vi "Arduino read multiple 11-08-2017 w median filt.vi"(7 "loop cycle in":u32=300, 8 "freq in":dbl[](array[numeric]), 10 "arduino addresses in":T2) -> (0 "loop cycle out":u32=300, 1 "freq out":dbl[](array[numeric]), 3 "arduino addresses out":T1)   [LabVIEW 2014]
uses:
  <vilib>/Analysis/NI_AALBase.lvlib
panel:
  out "median":dbl format="%0.2f"
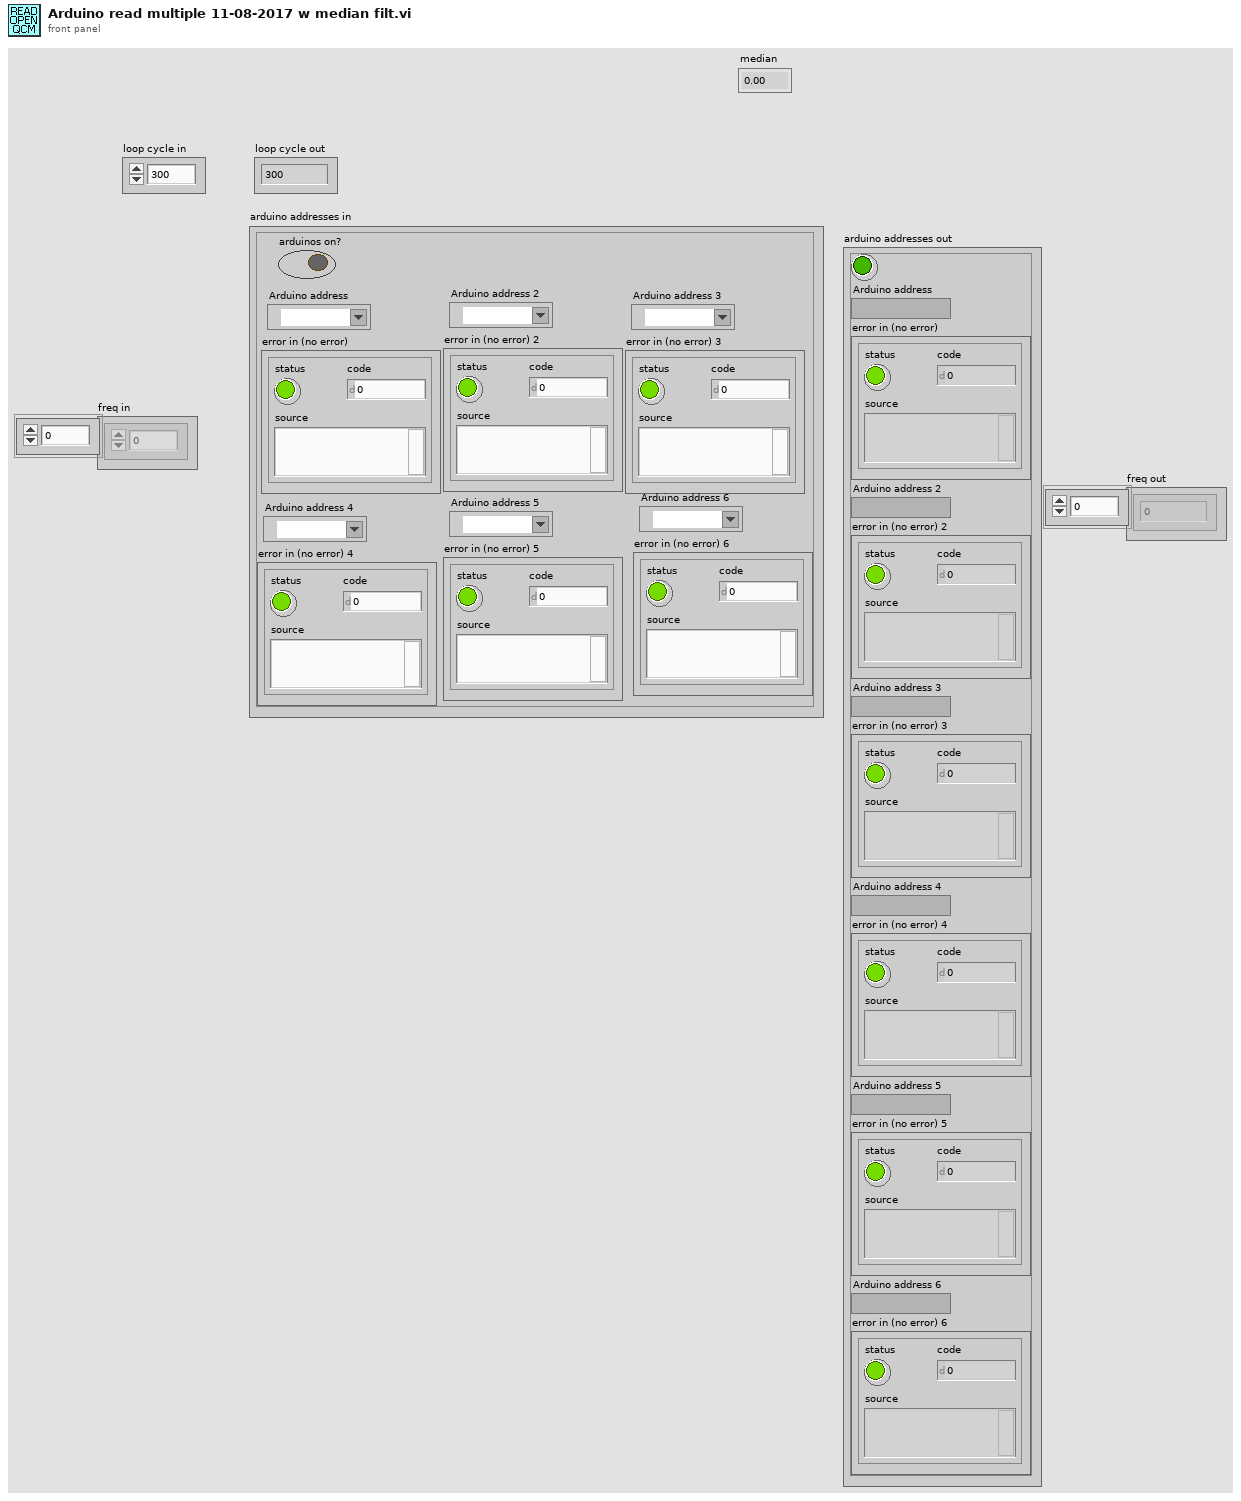
[diagram p1: front panel]
types:
  T1 = cluster{"Boolean":bool, "Arduino address":refnum<visa-resource-name>, "error in (no error)":errorcluster, "Arduino address 2":refnum<visa-resource-name>, "error in (no error) 2":errorcluster, "Arduino address 3":refnum<visa-resource-name>, "error in (no error) 3":errorcluster, "Arduino address 4":refnum<visa-resource-name>, "error in (no error) 4":errorcluster, "Arduino address 5":refnum<visa-resource-name>, "error in (no error) 5":errorcluster, "Arduino address 6":refnum<visa-resource-name>, "error in (no error) 6":errorcluster}
  T2 = cluster{"Arduino address":refnum<visa-resource-name>, "error in (no error)":errorcluster, "Arduino address 2":refnum<visa-resource-name>, "error in (no error) 2":errorcluster, "Arduino address 3":refnum<visa-resource-name>, "error in (no error) 3":errorcluster, "Arduino address 4":refnum<visa-resource-name>, "error in (no error) 4":errorcluster, "Arduino address 5":refnum<visa-resource-name>, "error in (no error) 5":errorcluster, "Arduino address 6":refnum<visa-resource-name>, "error in (no error) 6":errorcluster, "arduinos on?":bool}
  T3 = cluster{bool, "Arduino address":refnum<visa-resource-name>, "error in (no error)":errorcluster, "Arduino address 2":refnum<visa-resource-name>, "error in (no error) 2":errorcluster, "Arduino address 3":refnum<visa-resource-name>, "error in (no error) 3":errorcluster, "Arduino address 4":refnum<visa-resource-name>, "error in (no error) 4":errorcluster, "Arduino address 5":refnum<visa-resource-name>, "error in (no error) 5":errorcluster, "Arduino address 6":refnum<visa-resource-name>, "error in (no error) 6":errorcluster}
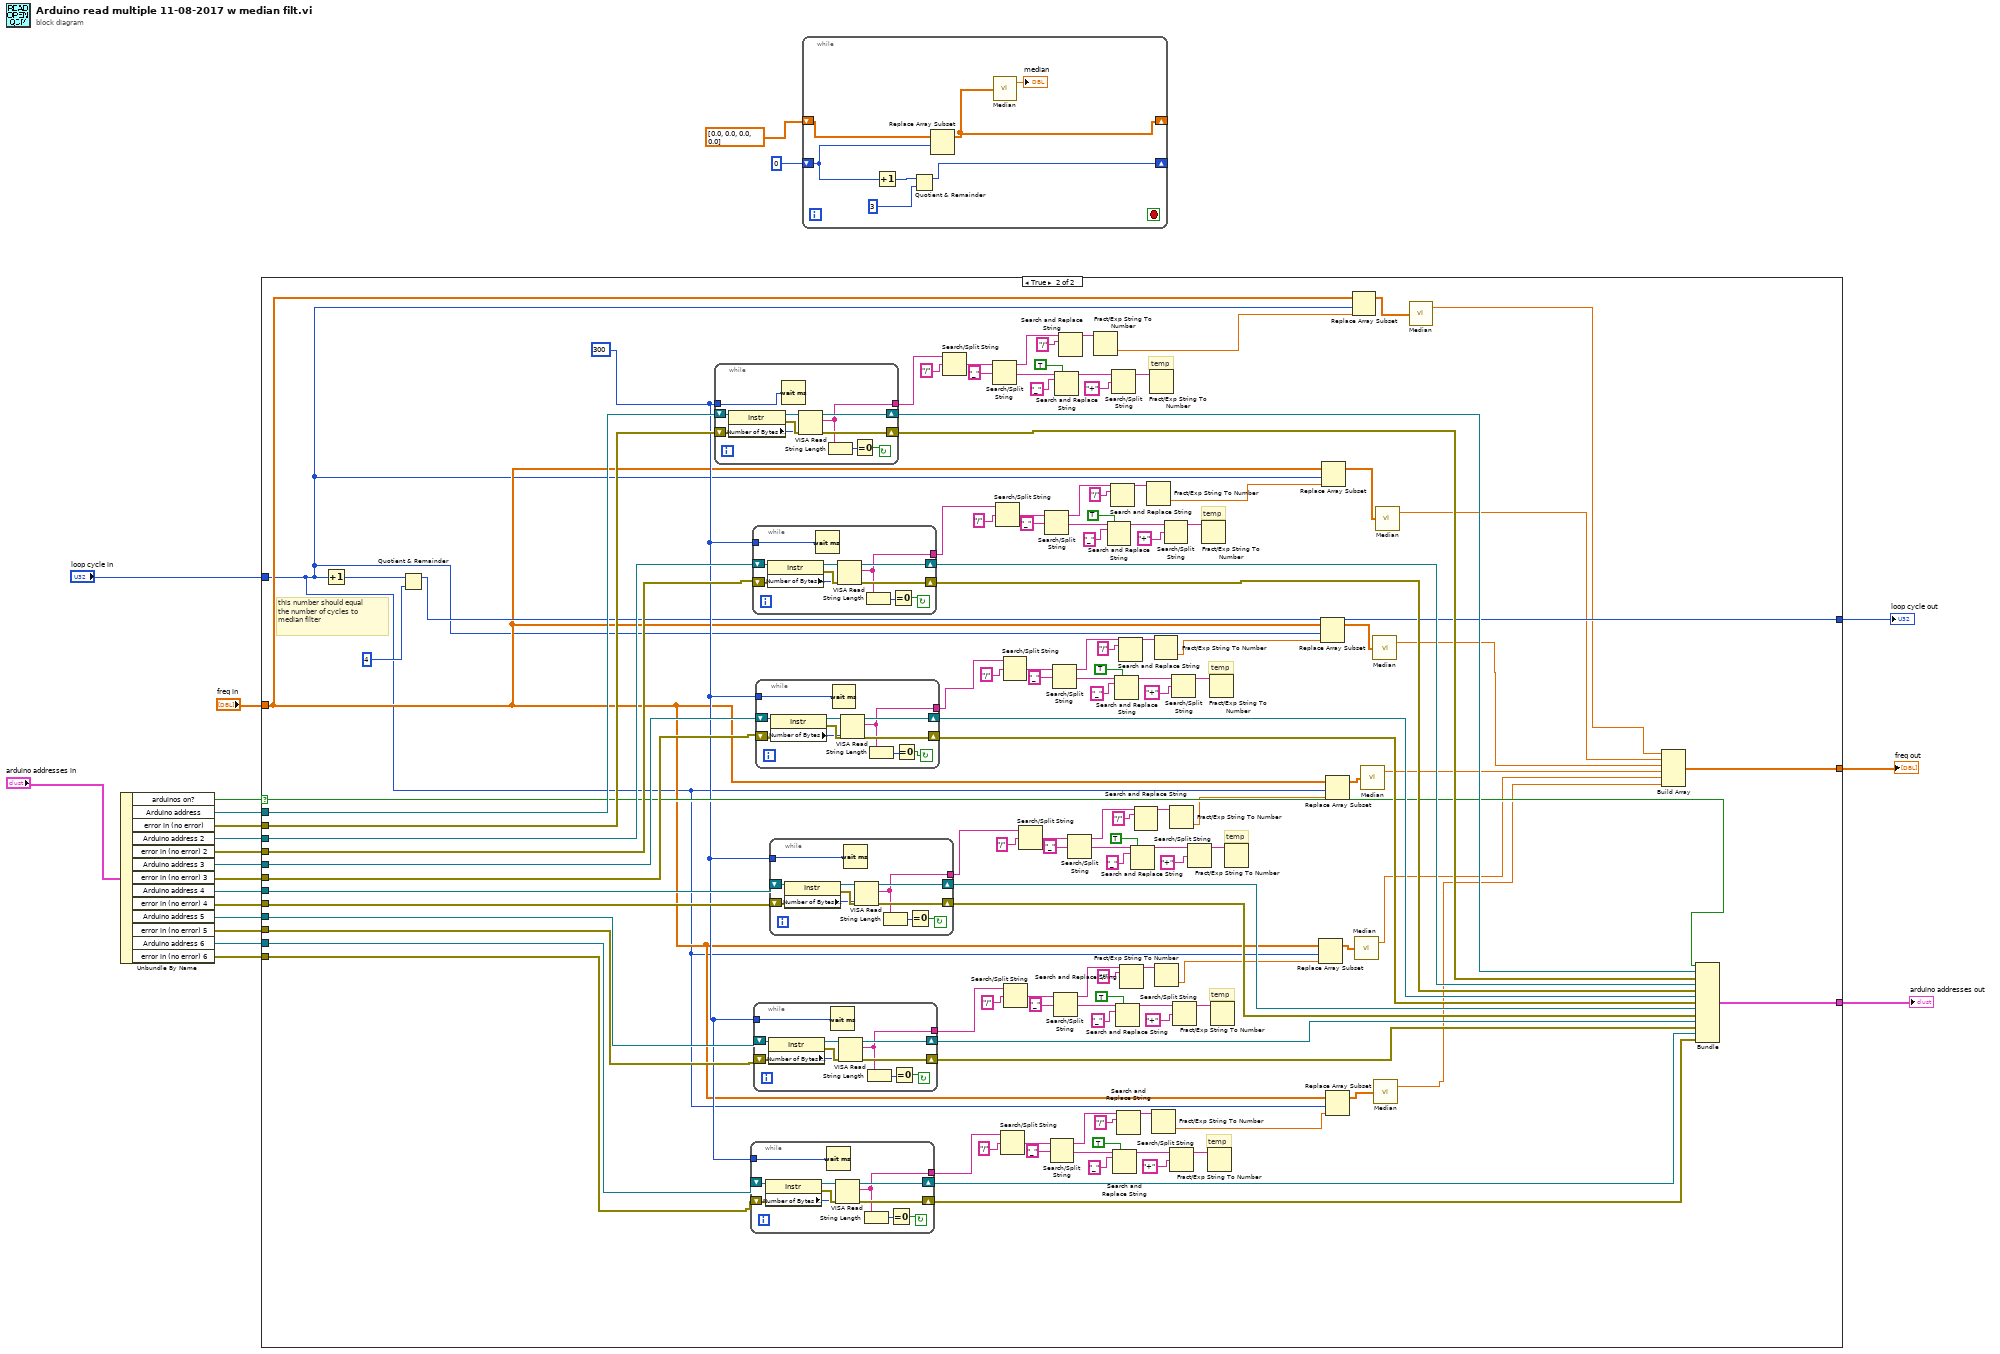
[diagram p0: block diagram]
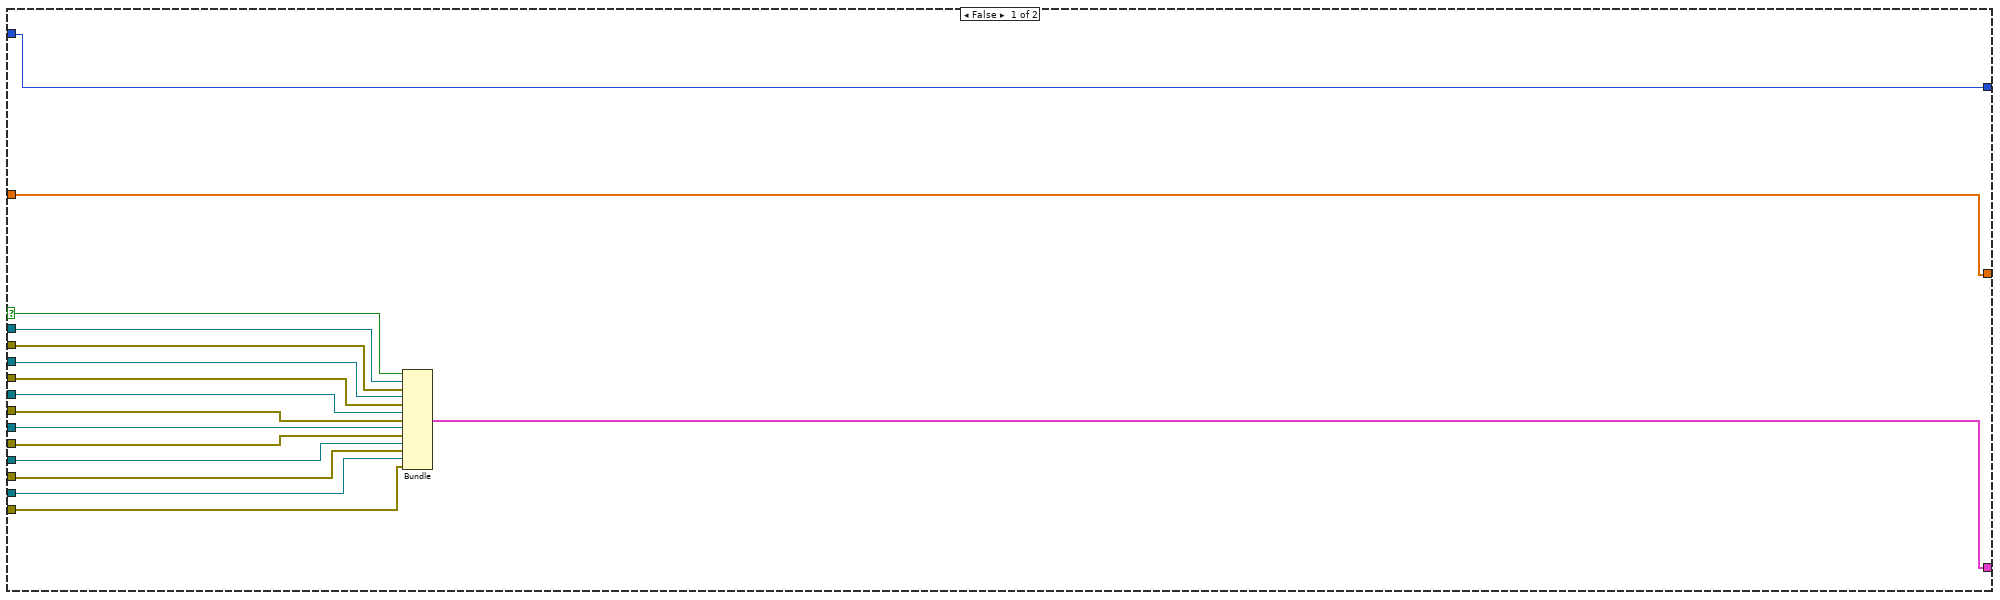
[diagram p2: hidden frame]
diagram:
  n1 = Unbundle By Name("arduino addresses in") -> ("arduinos on?"=w21:bool, "Arduino address"=w20:refnum<visa-resource-name>, "error in (no error)"=w19:errorcluster, "Arduino address 2"=w18:refnum<visa-resource-name>, "error in (no error) 2"=w17:errorcluster, "Arduino address 3"=w16:refnum<visa-resource-name>, "error in (no error) 3"=w15:errorcluster, "Arduino address 4"=w13:refnum<visa-resource-name>, "error in (no error) 4"=w12:errorcluster, "Arduino address 5"=w11:refnum<visa-resource-name>, "error in (no error) 5"=w10:errorcluster, "Arduino address 6"=w9:refnum<visa-resource-name>, "error in (no error) 6"=w8:errorcluster)
  n2 = case shown="True" w21 {
    selector: w21 -> [w37 w64]
    tunnel: [w22 w63] -> w7
    tunnel: w20 -> [w36 w76]
    tunnel: w19 -> [w35 w75]
    tunnel: w18 -> [w34 w74]
    tunnel: w17 -> [w33 w73]
    tunnel: w16 -> [w32 w72]
    tunnel: w15 -> [w31 w71]
    tunnel: w13 -> [w30 w70]
    tunnel: w12 -> [w29 w69]
    tunnel: w11 -> [w28 w68]
    tunnel: w10 -> [w27 w67]
    tunnel: w9 -> [w26 w66]
    tunnel: w8 -> [w25 w65]
    tunnel: [w23 w62] -> w6
    tunnel: "freq in" -> [w23 w57]
    tunnel: "loop cycle in" -> [w24 w56]
    tunnel: [w24 w58] -> w3
    frame False {
      n3 = Bundle(w37, "Arduino address"=w36, "error in (no error)"=w35, "Arduino address 2"=w34, "error in (no error) 2"=w33, "Arduino address 3"=w32, "error in (no error) 3"=w31, "Arduino address 4"=w30, "error in (no error) 4"=w29, "Arduino address 5"=w28, "error in (no error) 5"=w27, "Arduino address 6"=w26, "error in (no error) 6"=w25) -> (w22:T3)  [unwired: 1 in]
    }
    frame True {
      w61 = u32 300 ("milliseconds to wait")
      # "this number should equal the number of cycles to median filter"
      # "temp"
      # "temp"
      # "temp"
      # "temp"
      # "temp"
      # "temp"
      n4 = Increment(x=w56) -> (x+1=w59:u32)
      n5 = Quotient & Remainder(x=w59, y=u32 4 ("this number should equal the nubmer of cycles to take median over")) -> (x-y*floor(x/y)=w58:u32)  [unwired: 1 out]
      n6 = while {
        shift-right: [w232] -> w88
        shift-left: w76 -> [w230]
        shift-right: [w231] -> w87
        shift-left: w75 -> [w229]
        tunnel: [w223] -> w154
        tunnel: w61 -> [w222]
        stop <- w224 continue-if-true
        n7 = property class="Instr"(reference=w230, error in=w229) -> (reference out=w227:refnum<visa-resource-name>, error out=w228:errorcluster, "Serial Settings:Number of Bytes at Serial Port"=w226:u32)
        n8 = Wait (ms)(milliseconds to wait=w222) -> ()  [unwired: 1 out]
        n9 = VISA Read(VISA resource name=w227, byte count=w226, error in (no error)=w228) -> (VISA resource name out=w232:refnum<visa-resource-name>, read buffer=w223:string, error out=w231:errorcluster)  [unwired: 1 out]
        n10 = String Length(string=w223) -> (length=w225:i32)
        n11 = Equal To 0?(x=w225) -> (x = 0?=w224:bool)
      }
      n12 = while {
        shift-right: [w177] -> w79
        shift-left: w66 -> [w175]
        shift-right: [w176] -> w78
        shift-left: w65 -> [w174]
        tunnel: [w168] -> w89
        tunnel: w61 -> [w167]
        stop <- w169 continue-if-true
        n13 = property class="Instr"(reference=w175, error in=w174) -> (reference out=w172:refnum<visa-resource-name>, error out=w173:errorcluster, "Serial Settings:Number of Bytes at Serial Port"=w171:u32)
        n14 = Wait (ms)(milliseconds to wait=w167) -> ()  [unwired: 1 out]
        n15 = VISA Read(VISA resource name=w172, byte count=w171, error in (no error)=w173) -> (VISA resource name out=w177:refnum<visa-resource-name>, read buffer=w168:string, error out=w176:errorcluster)  [unwired: 1 out]
        n16 = String Length(string=w168) -> (length=w170:i32)
        n17 = Equal To 0?(x=w170) -> (x = 0?=w169:bool)
      }
      n18 = while {
        shift-right: [w221] -> w86
        shift-left: w74 -> [w219]
        shift-right: [w220] -> w85
        shift-left: w73 -> [w218]
        tunnel: [w212] -> w141
        tunnel: w61 -> [w211]
        stop <- w213 continue-if-true
        n19 = property class="Instr"(reference=w219, error in=w218) -> (reference out=w216:refnum<visa-resource-name>, error out=w217:errorcluster, "Serial Settings:Number of Bytes at Serial Port"=w215:u32)
        n20 = Wait (ms)(milliseconds to wait=w211) -> ()  [unwired: 1 out]
        n21 = VISA Read(VISA resource name=w216, byte count=w215, error in (no error)=w217) -> (VISA resource name out=w221:refnum<visa-resource-name>, read buffer=w212:string, error out=w220:errorcluster)  [unwired: 1 out]
        n22 = String Length(string=w212) -> (length=w214:i32)
        n23 = Equal To 0?(x=w214) -> (x = 0?=w213:bool)
      }
      n24 = while {
        shift-right: [w188] -> w77
        shift-left: w68 -> [w186]
        shift-right: [w187] -> w80
        shift-left: w67 -> [w185]
        tunnel: [w179] -> w102
        tunnel: w61 -> [w178]
        stop <- w180 continue-if-true
        n25 = property class="Instr"(reference=w186, error in=w185) -> (reference out=w183:refnum<visa-resource-name>, error out=w184:errorcluster, "Serial Settings:Number of Bytes at Serial Port"=w182:u32)
        n26 = Wait (ms)(milliseconds to wait=w178) -> ()  [unwired: 1 out]
        n27 = VISA Read(VISA resource name=w183, byte count=w182, error in (no error)=w184) -> (VISA resource name out=w188:refnum<visa-resource-name>, read buffer=w179:string, error out=w187:errorcluster)  [unwired: 1 out]
        n28 = String Length(string=w179) -> (length=w181:i32)
        n29 = Equal To 0?(x=w181) -> (x = 0?=w180:bool)
      }
      n30 = while {
        shift-right: [w210] -> w84
        shift-left: w72 -> [w208]
        shift-right: [w209] -> w83
        shift-left: w71 -> [w207]
        tunnel: [w201] -> w128
        tunnel: w61 -> [w200]
        stop <- w202 continue-if-true
        n31 = property class="Instr"(reference=w208, error in=w207) -> (reference out=w205:refnum<visa-resource-name>, error out=w206:errorcluster, "Serial Settings:Number of Bytes at Serial Port"=w204:u32)
        n32 = Wait (ms)(milliseconds to wait=w200) -> ()  [unwired: 1 out]
        n33 = VISA Read(VISA resource name=w205, byte count=w204, error in (no error)=w206) -> (VISA resource name out=w210:refnum<visa-resource-name>, read buffer=w201:string, error out=w209:errorcluster)  [unwired: 1 out]
        n34 = String Length(string=w201) -> (length=w203:i32)
        n35 = Equal To 0?(x=w203) -> (x = 0?=w202:bool)
      }
      n36 = while {
        shift-right: [w199] -> w82
        shift-left: w70 -> [w197]
        shift-right: [w198] -> w81
        shift-left: w69 -> [w196]
        tunnel: [w190] -> w115
        tunnel: w61 -> [w189]
        stop <- w191 continue-if-true
        n37 = property class="Instr"(reference=w197, error in=w196) -> (reference out=w194:refnum<visa-resource-name>, error out=w195:errorcluster, "Serial Settings:Number of Bytes at Serial Port"=w193:u32)
        n38 = Wait (ms)(milliseconds to wait=w189) -> ()  [unwired: 1 out]
        n39 = VISA Read(VISA resource name=w194, byte count=w193, error in (no error)=w195) -> (VISA resource name out=w199:refnum<visa-resource-name>, read buffer=w190:string, error out=w198:errorcluster)  [unwired: 1 out]
        n40 = String Length(string=w190) -> (length=w192:i32)
        n41 = Equal To 0?(x=w192) -> (x = 0?=w191:bool)
      }
      n42 = Search/Split String(string=w154, search string/char (-)="/") -> (match + rest of string=w160:string)  [unwired: 1 in, 2 out]
      n43 = Search/Split String(string=w160, search string/char (-)="_") -> (substring before match=w166:string, match + rest of string=w161:string)  [unwired: 1 in, 1 out]
      n44 = Search/Split String(string=w141, search string/char (-)="/") -> (match + rest of string=w147:string)  [unwired: 1 in, 2 out]
      n45 = Search/Split String(string=w89, search string/char (-)="/") -> (match + rest of string=w95:string)  [unwired: 1 in, 2 out]
      n46 = Search/Split String(string=w128, search string/char (-)="/") -> (match + rest of string=w134:string)  [unwired: 1 in, 2 out]
      n47 = Search/Split String(string=w102, search string/char (-)="/") -> (match + rest of string=w108:string)  [unwired: 1 in, 2 out]
      n48 = Search/Split String(string=w115, search string/char (-)="/") -> (match + rest of string=w121:string)  [unwired: 1 in, 2 out]
      n49 = Search/Split String(string=w147, search string/char (-)="_") -> (substring before match=w153:string, match + rest of string=w148:string)  [unwired: 1 in, 1 out]
      n50 = Search/Split String(string=w95, search string/char (-)="_") -> (substring before match=w101:string, match + rest of string=w96:string)  [unwired: 1 in, 1 out]
      n51 = Search/Split String(string=w134, search string/char (-)="_") -> (substring before match=w140:string, match + rest of string=w135:string)  [unwired: 1 in, 1 out]
      n52 = Search/Split String(string=w108, search string/char (-)="_") -> (substring before match=w114:string, match + rest of string=w109:string)  [unwired: 1 in, 1 out]
      n53 = Search and Replace String(replace all?=TRUE ("replace all? (F)"), input string=w161, search string="_") -> (result string=w155:string)  [unwired: 5 in, 3 out]
      n54 = Search and Replace String(input string=w166, search string="/" ("replace string (\"\")")) -> (result string=w157:string)  [unwired: 6 in, 3 out]
      n55 = Search/Split String(string=w121, search string/char (-)="_") -> (substring before match=w127:string, match + rest of string=w122:string)  [unwired: 1 in, 1 out]
      n56 = Fract/Exp String To Number(string=w157) -> (number=w55:dbl)  [unwired: 3 in, 1 out]
      n57 = Search and Replace String(replace all?=TRUE ("replace all? (F)"), input string=w148, search string="_") -> (result string=w142:string)  [unwired: 5 in, 3 out]
      n58 = Search and Replace String(input string=w153, search string="/" ("replace string (\"\")")) -> (result string=w144:string)  [unwired: 6 in, 3 out]
      n59 = Search/Split String(string=w155, search string/char (-)="+") -> (substring before match=w164:string)  [unwired: 1 in, 2 out]
      n60 = Search and Replace String(replace all?=TRUE ("replace all? (F)"), input string=w96, search string="_") -> (result string=w90:string)  [unwired: 5 in, 3 out]
      n61 = Search and Replace String(replace all?=TRUE ("replace all? (F)"), input string=w135, search string="_") -> (result string=w129:string)  [unwired: 5 in, 3 out]
      n62 = Search and Replace String(replace all?=TRUE ("replace all? (F)"), input string=w109, search string="_") -> (result string=w103:string)  [unwired: 5 in, 3 out]
      n63 = Search and Replace String(input string=w101, search string="/" ("replace string (\"\")")) -> (result string=w92:string)  [unwired: 6 in, 3 out]
      n64 = Search and Replace String(input string=w140, search string="/" ("replace string (\"\")")) -> (result string=w131:string)  [unwired: 6 in, 3 out]
      n65 = Search and Replace String(input string=w114, search string="/" ("replace string (\"\")")) -> (result string=w105:string)  [unwired: 6 in, 3 out]
      n66 = Search and Replace String(replace all?=TRUE ("replace all? (F)"), input string=w122, search string="_") -> (result string=w116:string)  [unwired: 5 in, 3 out]
      n67 = Search and Replace String(input string=w127, search string="/" ("replace string (\"\")")) -> (result string=w118:string)  [unwired: 6 in, 3 out]
      n68 = Fract/Exp String To Number(string=w144) -> (number=w52:dbl)  [unwired: 3 in, 1 out]
      n69 = Fract/Exp String To Number(string=w164) -> ()  [unwired: 3 in, 2 out]
      n70 = Fract/Exp String To Number(string=w92) -> (number=w40:dbl)  [unwired: 3 in, 1 out]
      n71 = Fract/Exp String To Number(string=w131) -> (number=w49:dbl)  [unwired: 3 in, 1 out]
      n72 = Fract/Exp String To Number(string=w105) -> (number=w43:dbl)  [unwired: 3 in, 1 out]
      n73 = Search/Split String(string=w142, search string/char (-)="+") -> (substring before match=w151:string)  [unwired: 1 in, 2 out]
      n74 = Fract/Exp String To Number(string=w118) -> (number=w46:dbl)  [unwired: 3 in, 1 out]
      n75 = Search/Split String(string=w90, search string/char (-)="+") -> (substring before match=w99:string)  [unwired: 1 in, 2 out]
      n76 = Search/Split String(string=w129, search string/char (-)="+") -> (substring before match=w138:string)  [unwired: 1 in, 2 out]
      n77 = Search/Split String(string=w103, search string/char (-)="+") -> (substring before match=w112:string)  [unwired: 1 in, 2 out]
      n78 = Search/Split String(string=w116, search string/char (-)="+") -> (substring before match=w125:string)  [unwired: 1 in, 2 out]
      n79 = Fract/Exp String To Number(string=w151) -> ()  [unwired: 3 in, 2 out]
      n80 = Fract/Exp String To Number(string=w99) -> ()  [unwired: 3 in, 2 out]
      n81 = Fract/Exp String To Number(string=w138) -> ()  [unwired: 3 in, 2 out]
      n82 = Fract/Exp String To Number(string=w112) -> ()  [unwired: 3 in, 2 out]
      n83 = Fract/Exp String To Number(string=w125) -> ()  [unwired: 3 in, 2 out]
      n84 = Replace Array Subset(array=w57, new element=w43, index=w56) -> (w42:dbl[])
      n85 = Replace Array Subset(array=w57, new element=w49, index=w56) -> (w48:dbl[])
      n86 = Replace Array Subset(array=w57, new element=w52, index=w56) -> (w51:dbl[])
      n87 = Replace Array Subset(array=w57, new element=w46, index=w56) -> (w45:dbl[])
      n88 = Replace Array Subset(array=w57, new element=w40, index=w56) -> (w39:dbl[])
      n89 = Replace Array Subset(array=w57, new element=w55, index=w56) -> (w54:dbl[])
      n90 = call <vilib>:"Median.vi"("X"=w42) -> ("median"=w41:dbl)  [unwired: 1 out]
      n91 = call <vilib>:"Median.vi"("X"=w45) -> ("median"=w44:dbl)  [unwired: 1 out]
      n92 = call <vilib>:"Median.vi"("X"=w48) -> ("median"=w47:dbl)  [unwired: 1 out]
      n93 = call <vilib>:"Median.vi"("X"=w39) -> ("median"=w38:dbl)  [unwired: 1 out]
      n94 = call <vilib>:"Median.vi"("X"=w51) -> ("median"=w50:dbl)  [unwired: 1 out]
      n95 = call <vilib>:"Median.vi"("X"=w54) -> ("median"=w53:dbl)  [unwired: 1 out]
      n96 = Build Array(w53, w50, w47, w44, w41, w38) -> (w62:dbl[])
      n97 = Bundle(w64, "Arduino address"=w88, "error in (no error)"=w87, "Arduino address 2"=w86, "error in (no error) 2"=w85, "Arduino address 3"=w84, "error in (no error) 3"=w83, "Arduino address 4"=w82, "error in (no error) 4"=w81, "Arduino address 5"=w77, "error in (no error) 5"=w80, "Arduino address 6"=w79, "error in (no error) 6"=w78) -> (w63:T3)  [unwired: 1 in]
    }
  }
  "arduino addresses out" <- w7
  "freq out" <- w6
  "loop cycle out" <- w3
  n98 = while {
    shift-right: [w233] -> _
    shift-left: u32 0 ("loop cycle in 2") -> [w235]
    shift-right: [w236] -> _
    shift-left: dbl[] [0.0, 0.0, 0.0, 0.0] ("freq in 3") -> [w237]
    stop <- _ stop-if-true
    n99 = Increment(x=w235) -> (x+1=w238:u32)
    n100 = Quotient & Remainder(x=w238, y=u32 3 ("this number should equal the nubmer of cycles to take median over")) -> (x-y*floor(x/y)=w233:u32)  [unwired: 1 out]
    n101 = Replace Array Subset(array=w237, index=w235) -> (w236:dbl[])  [unwired: 1 in]
    n102 = call <vilib>:"Median.vi"("X"=w236) -> ("median"=→"median":dbl)  [unwired: 1 out]
  }
